vi "__Update Drive List.vi"(8 "error in (no error)":errorcluster, 11 "FileManager Ctl Refs in":T1) -> (0 "error out":errorcluster, 3 "FileManager Ctl Refs out":T1)   [LabVIEW 2011]
doc: "Requests the drive letters available on the local system and then populates the Local Drives ComboBox on the application front panel with the values."
uses:
  __File manager Data type.ctl
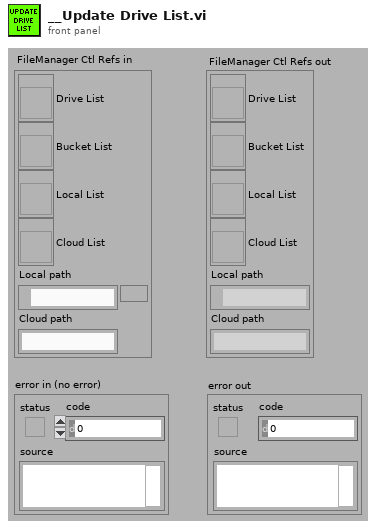
[diagram p1: front panel]
types:
  T1 = typedef "__File manager Data type.ctl" = cluster{"Drive List":refnum<vi>, "Bucket List":refnum<vi>, "Local List":refnum<vi>, "Cloud List":refnum<vi>, "Local path":path, "Cloud path":string}
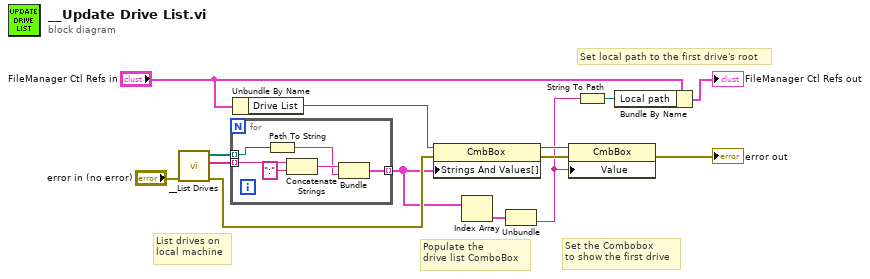
[diagram p0: block diagram]
diagram:
  # "Set local path to the first drive's root"
  # "Set the Combobox\nto show the first drive"
  # "Populate the\ndrive list ComboBox"
  # "List drives on\nlocal machine"
  n1 = call "__List Drives.vi"("error in (no error)"="error in (no error)") -> ("error out"=w11:errorcluster, "Drive letters"=w12:string[], "Drive paths"=w13:path[])  [unwired: 8 in]
  n2 = for {
    tunnel: w13 -> [w17] mode=indexing
    tunnel: w12 -> [w20] mode=indexing
    tunnel: [w15] -> w7 mode=indexing
    n3 = Path To String(path=w17) -> (string=w16:string)
    n4 = Concatenate Strings(w20, ":" ("string")) -> (w18:string)
    n5 = Bundle(w18, w16) -> (w15:cluster{string, string})  [unwired: 1 in]
  }
  n6 = Unbundle By Name("FileManager Ctl Refs in") -> ("Drive List"=w5:refnum<vi>)
  n7 = property class="CmbBox"(reference=w5, error in=w11, "Strings And Values[]"=w7) -> (reference out=w8:refnum<vi>, error out=w9:errorcluster)
  n8 = Index Array(array=w7) -> (element=w6:cluster{string, string})  [unwired: 1 in]
  n9 = Unbundle(w6) -> (w2:string)  [unwired: 1 out]
  n10 = property class="CmbBox"(reference=w8, error in=w9, "Value"=w2) -> (error out=→"error out":errorcluster)  [unwired: 1 out]
  n11 = String To Path(string=w2) -> (path=w1:path)
  n12 = Bundle By Name(cluster="FileManager Ctl Refs in", "Local path"=w1) -> (→"FileManager Ctl Refs out":T1)
